vi "UI_ShowIn_Subpanel.vi"(8 "error in (no error)":errorcluster, 10 "Sub Panel":refnum<vi>, 11 "DualScreen in":refnum<class "DualScreen.lvclass">) -> (0 "error out":errorcluster, 3 "DualScreen out":refnum<class "DualScreen.lvclass">)   [LabVIEW 2020, in "DualScreen.lvlib" / "DualScreen.lvclass"]
uses:
  DualScreen.lvclass
  D:/Projets/STEP AT/Bahamut/support/UI_Actor.lvlibp/UI_Actor/UI_Actor.lvclass
  DualScreen.lvclass/DualScreen.ctl
  support/UI_Actor.lvlibp/UI_Actor/Read Nested UIA Qs.vi
  D&C_SchemaBase/D&C_SchemaBase/D&C_SchemaBase.lvclass
  support/Actor Framework.lvlibp/1abvi3w/vi.lib/ActorFramework/Message Enqueuer/Message Enqueuer.lvclass
  support/UI_Actor.lvlibp/UI_Actor Messages/UI_ShowIn_Subpanel Msg/UI_ShowIn_Subpanel Msg.lvclass
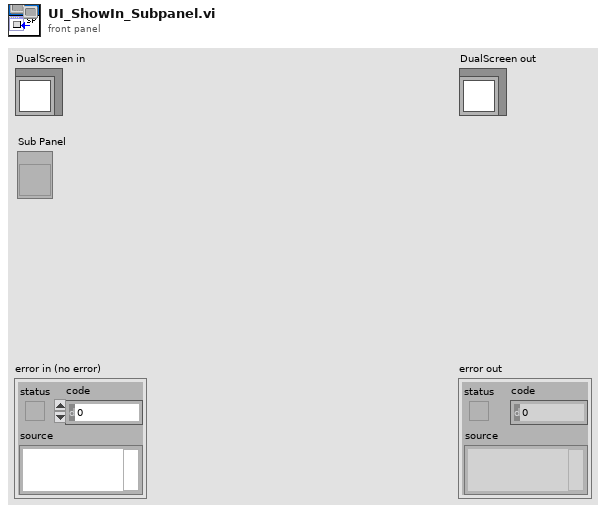
[diagram p1: front panel]
types:
  T1 = enum16{"Sticks Top/Left", "Sticks Bottom/Right", "Proportional"}
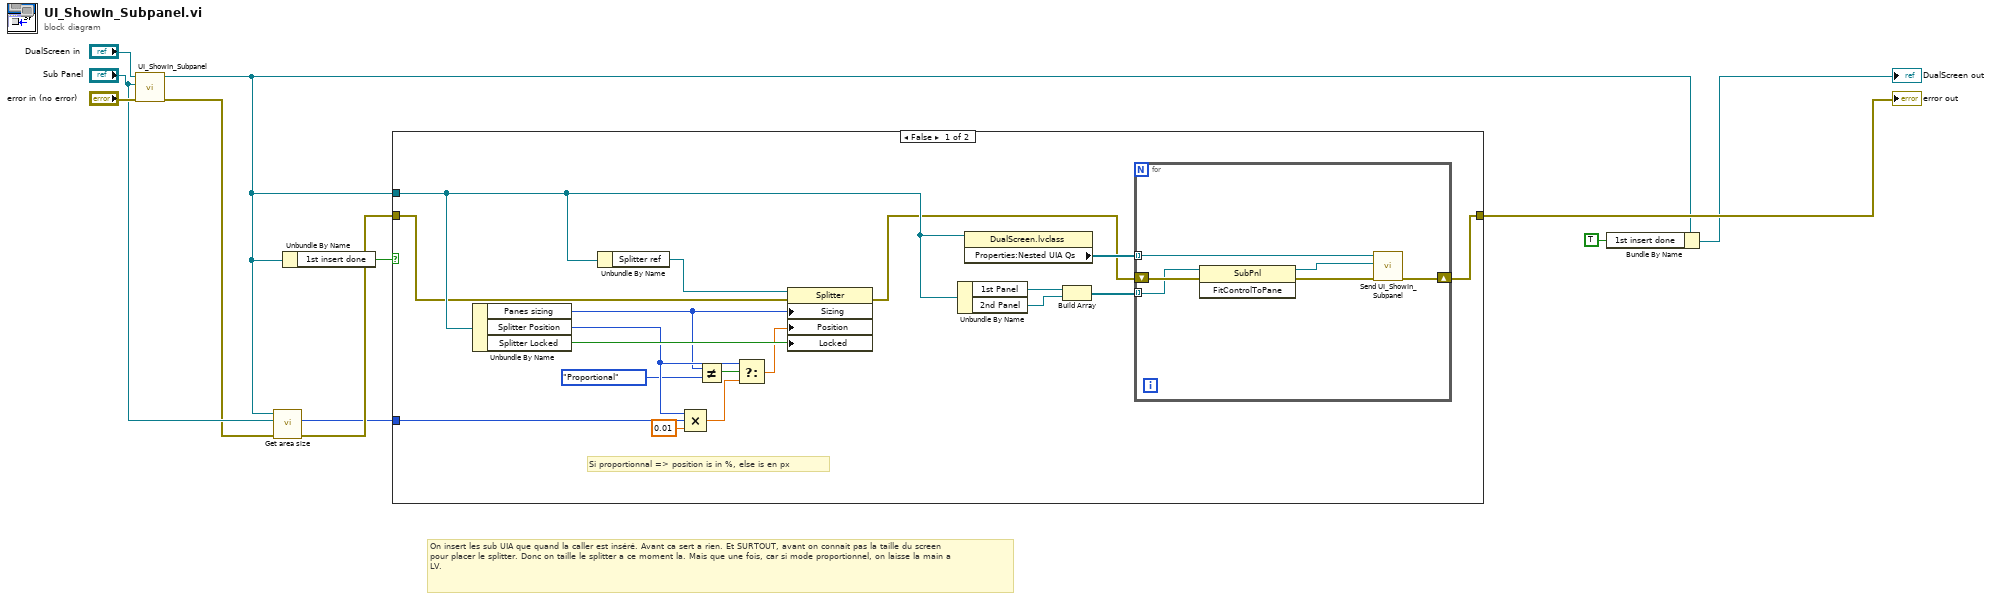
[diagram p0: block diagram]
diagram:
  # "On insert les sub UIA que quand la caller est inséré. Avant ca sert a rien. Et SURTOUT, avant on connait pas la taille du screen pour placer le splitter. Donc on taille le splitter a ce moment la. Mais que une fois, car si mode proportionnel, on laisse la main a LV."
  n1 = call-parent "UI_ShowIn_Subpanel.vi"("error in (no error)"="error in (no error)", "Sub Panel"="Sub Panel", "D&C_SchemaBase in"="DualScreen in") -> ("error out"=w3:errorcluster, "D&C_SchemaBase out"=w4:refnum<class "DualScreen.lvclass">)  [unwired: 7 in]
  n2 = call-dynamic "Get area size.vi"("error in (no error)"=w3, "Sub Panel"="Sub Panel", "DualScreen in"=w4) -> ("error out"=w2:errorcluster, "Area size (px)"=w1:u32)  [unwired: 6 in, 1 out]
  n3 = Unbundle By Name(w4) -> ("1st insert done"=w8:bool)
  n4 = case shown="False" w8 {
    tunnel: w2 -> [w14 w36]
    tunnel: [w26 w36] -> w7
    tunnel: w4 -> [w16 _]
    tunnel: w1 -> [w13 _]
    frame False {
      # "Si proportionnal => position is in %, else is en px"
      n5 = Unbundle By Name(w16) -> ("Panes sizing"=w20:T1, "Splitter Position"=w24:i32, "Splitter Locked"=w25:bool)
      n6 = Unbundle By Name(w16) -> ("Splitter ref"=w17:refnum<vi>)
      n7 = Compound Arithmetic op=MULTIPLY(w24, w13, 0.01 ("value")) -> (w23:dbl)
      n8 = Not Equal?(x=w20, y=T1."Proportional") -> (x != y?=w21:bool)
      n9 = Select(t=w24, s=w21, f=w23) -> (s? t:f=w22:dbl)
      n10 = property class="Splitter"(reference=w17, error in=w14, "Sizing"=w20, "Position"=w22, "Locked"=w25) -> (error out=w15:errorcluster)  [unwired: 1 out]
      n11 = Unbundle By Name(w16) -> ("1st Panel"=w12:refnum<vi>, "2nd Panel"=w28:refnum<vi>)
      n12 = property class="DualScreen.lvclass"(reference=w16) -> ("Properties:Nested UIA Qs"=w29:refnum<class "Message Enqueuer.lvclass">[])  [unwired: 1 in, 2 out]
      n13 = Build Array(w12, w28) -> (w27:refnum<vi>[])
      n14 = for {
        tunnel: w29 -> [w35] mode=indexing
        tunnel: w27 -> [w30] mode=indexing
        shift-right: [w34] -> w26
        shift-left: w15 -> [w33]
        n15 = invoke class="SubPnl" method="FitControlToPane"(reference=w30, error in=w33) -> (reference out=w31:refnum<vi>, error out=w32:errorcluster)  [unwired: 1 in, 1 out]
        n16 = call "Send UI_ShowIn_Subpanel.vi"("error in (no error)"=w32, "Sub Panel"=w31, "Message Enqueuer"=w35) -> ("error out"=w34:errorcluster)  [unwired: 7 in, 1 out]
      }
    }
    frame True {
    }
  }
  "error out" <- w7
  n17 = Bundle By Name(cluster=w4, "1st insert done"=TRUE ("1st resize done")) -> (→"DualScreen out":refnum<class "DualScreen.lvclass">)
